vi "Write Encryption.vi"(8 "error in (no error)":errorcluster, 10 "TSC Event Logger.lvlib:Encryption.lvclass":refnum<class "Encryption.lvclass">, 11 "Log Sinks in":refnum<class "Log Sinks.lvclass">) -> (0 "error out":errorcluster, 3 "Log Sinks out":refnum<class "Log Sinks.lvclass">)   [LabVIEW 2019, in "TSC Event Logger.lvlib" / "Log Sinks.lvclass"]
doc: "Data member access method to write the encryption type.\n\n<b>Code Developed By:</b>\nTechnology Service Corporation\nBloomington, IN 47403\nwww.tsc.com/atcs\n\nDeveloper:\nDaniel Coons"
uses:
  Log Sinks.lvclass
  Encryption/Encryption.lvclass
  Log Sinks.lvclass/Log Sinks.ctl
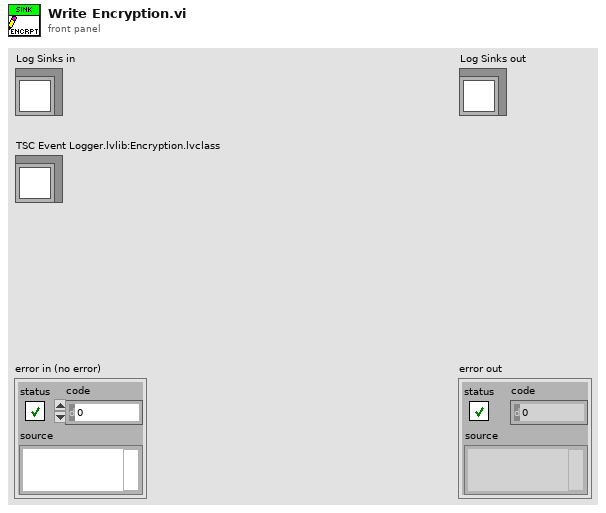
[diagram p1: front panel]
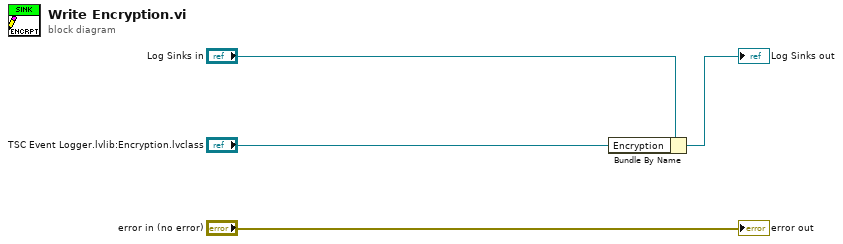
[diagram p0: block diagram]
diagram:
  n1 = Bundle By Name(cluster="Log Sinks in", "Encryption"="TSC Event Logger.lvlib:Encryption.lvclass") -> (→"Log Sinks out":refnum<class "Log Sinks.lvclass">)
  "error out" <- "error in (no error)"
